vi "AutoCorrelation Matrix (CDB).vi"(7 "initial?":bool, 9 "method":T1 items=["AutoCorrelation", "PreWindowed", "PostWindowed", "Covariance", "Modified Covariance"], 10 "order":i32, 11 "X":cdb[](array[numeric])) -> (0 "error":i32, 3 "AutoCorrelation Matrix":T2)   [LabVIEW 2017, in "NI_AAL_SigProc.lvlib"]
doc: "Computes the autocorrelation matrix of the input sequence <B>X</B>. Wire data to the <B>X</B> input to determine the polymorphic instance to use or manually select the instance."
uses:
  <vilib>/Analysis/NI_AAL_SigProc.lvlib
  <vilib>/Analysis/Matrix/Datatypes/ComplexMatrix.ctl
  <vilib>/Analysis/2dsp.llb/AutoCorrelation Matrix Method.ctl
  <resource>/lvanlys.dll
  <vilib>/Analysis/Matrix/NI_Matrix.lvlib
panel:
  # "AutoCorrelation Matrix (CDB)"
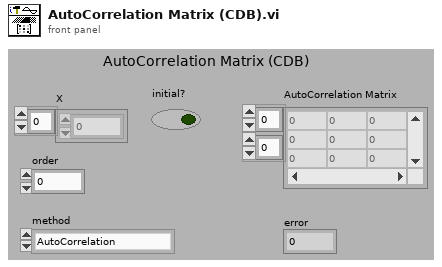
[diagram p1: front panel]
types:
  T1 = typedef "NI_AAL_SigProc.lvlib/AutoCorrelation Matrix Method.ctl" = i32
  T2 = typedef "NI_Matrix.lvlib/ComplexMatrix.ctl" = cdb[][]
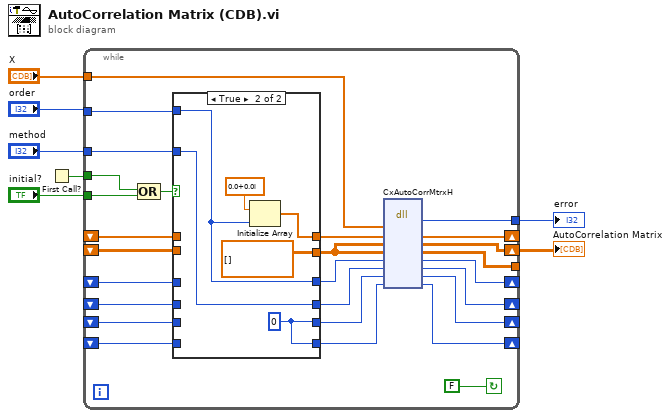
[diagram p0: block diagram]
diagram:
  n1 = First Call?() -> (First Call?: T/F=w1:bool)
  n2 = while {
    tunnel: "X" -> [w31]
    tunnel: "order" -> [w21]
    tunnel: "method" -> [w17]
    shift-right: [w30] -> w4
    shift-left: _ -> [w23]
    tunnel: [w29] -> w3
    shift-right: [w28] -> _
    shift-left: _ -> [w25]
    tunnel: "initial?" -> [w27]
    tunnel: [w22] -> _
    shift-right: [w19] -> _
    shift-left: _ -> [w18]
    shift-right: [w9] -> _
    shift-left: _ -> [w16]
    shift-right: [w10] -> _
    shift-left: _ -> [w15]
    shift-right: [w13] -> _
    shift-left: _ -> [w12]
    tunnel: w1 -> [w8]
    stop <- FALSE continue-if-true
    n3 = Compound Arithmetic op=OR(w8, w27) -> (w26:bool)
    n4 = case shown="True" w26 {
      tunnel: w25 -> [w37 _]
      tunnel: [w37 w43] -> w24
      tunnel: w23 -> [w36 _]
      tunnel: [w36 T2 [] ("AutoCorrelation Matrix 2")] -> w11
      tunnel: w21 -> [_ w41]
      tunnel: [w38 w40] -> w20
      tunnel: w18 -> [w38 _]
      tunnel: w17 -> [_ w42]
      tunnel: [w33 w42] -> w9
      tunnel: w16 -> [w33 _]
      tunnel: [w35 w41] -> w10
      tunnel: w15 -> [w35 _]
      tunnel: [w34 w40] -> w14
      tunnel: w12 -> [w34 _]
      frame False {
      }
      frame True {
        w40 = 0 ("order")
        n5 = Initialize Array(cdb 0.0+0.0i ("element"), w41) -> (w43:cdb[])
      }
    }
    n6 = dll-call lib="e:/builds/penguin/labview/branches/2017/dev/dist/resource/lvanlys.*" fn="CxAutoCorrMtrxH"("X"=w31, "History"=w24, "AutoCorrMtrx"=w11, "Matrix_X"=w11, "order"=w10, "method"=w9, "index"=w20, "PrevSize"=w14) -> ("error"=w29:i32, "History"=w28:cdb[], "AutoCorrMtrx"=w30:T2, "Matrix_X"=w22:T2, "index"=w19:i32, "PrevSize"=w13:i32)  [unwired: 6 in, 2 out]
  }
  "AutoCorrelation Matrix" <- w4
  "error" <- w3
